vi "Vesta Communication.vi"(8 "error in (no error)":errorcluster, 11 "Message Queues out":T2) -> (0 "error out":errorcluster)   [LabVIEW 2023]
uses:
  Message Queue/All Message Queues.ctl
  Message Queue/Message Cluster.ctl
  Drivers/Resideo Gas Valve/Type Definitions/Vesta Info.ctl
  Drivers/Resideo Gas Valve/Type Definitions/Temperature Control.ctl
  Message Queue/Enqueue Message (Single).vi
  Message Queue/Message Queue.lvlib
panel:
  out "Vesta Data Output":T1
  in  "Debug":bool
  out "Debug":string[](array[string])
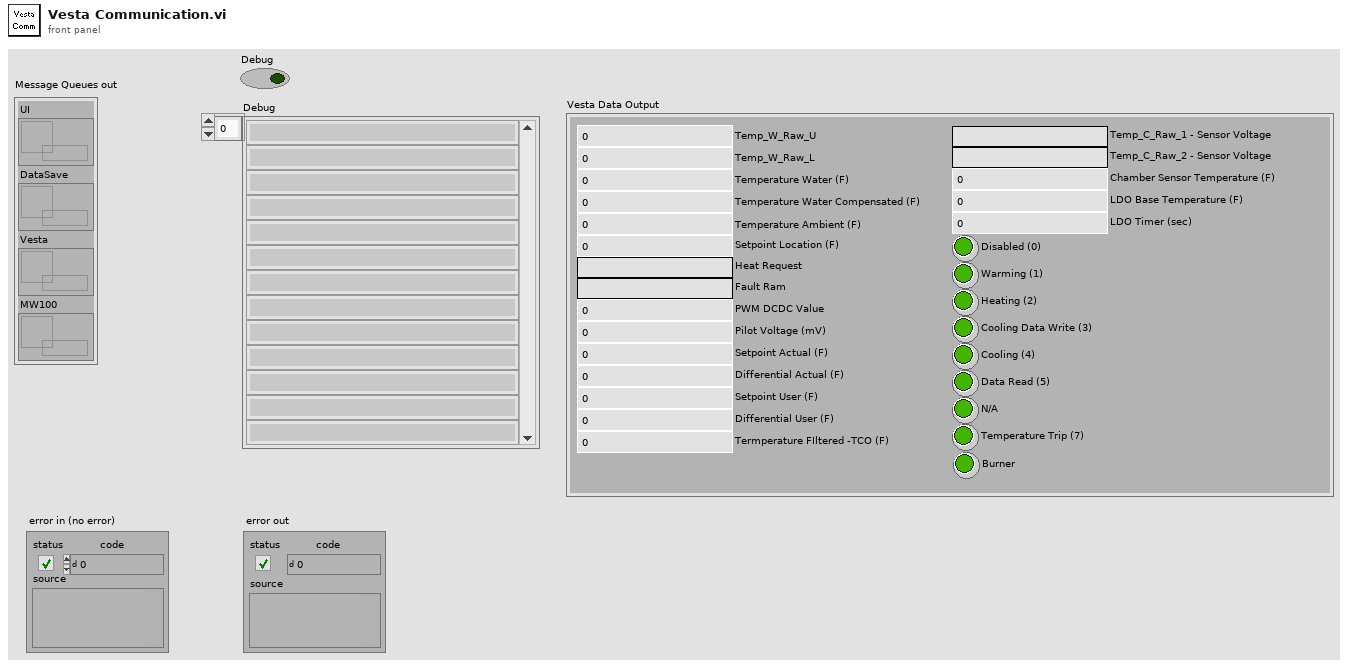
[diagram p1: front panel]
types:
  T1 = typedef "Vesta Info.ctl" = cluster{"Temp_W_Raw_U":u16, "Temp_W_Raw_L":u16, "Temperature Water (F)":dbl, "Temperature Water Compensated (F)":dbl, "Temperature Ambient (F)":dbl, "Setpoint Location (F)":dbl, "Heat Request":string, "Fault Ram":string, "PWM DCDC Value":u16, "Pilot Voltage (mV)":dbl, "Setpoint Actual (F)":dbl, "Differential Actual (F)":dbl, "Setpoint User (F)":dbl, "Differential User (F)":dbl, "Termperature FIltered -TCO (F)":dbl, "Temp_C_Raw_1 - Sensor Voltage":string, "Temp_C_Raw_2 - Sensor Voltage":string, "Chamber Sensor Temperature (F)":dbl, "LDO Base Temperature (F)":dbl, "LDO Timer (sec)":i16, "Disabled (0)":bool, "Warming (1)":bool, "Heating (2)":bool, "Cooling Data Write (3)":bool, "Cooling (4)":bool, "Data Read (5)":bool, "N/A":bool, "Temperature Trip (7)":bool, "Burner":bool}
  T2 = typedef "Message Queue.lvlib/All Message Queues.ctl" = cluster{"UI":refnum<queue>, "DataSave":refnum<queue>, "Vesta":refnum<queue>, "MW100":refnum<queue>}
  T3 = typedef "Temperature Control.ctl" = cluster{"Water Heater Temp (°F)":u16, "Differential  (°F)":dbl}
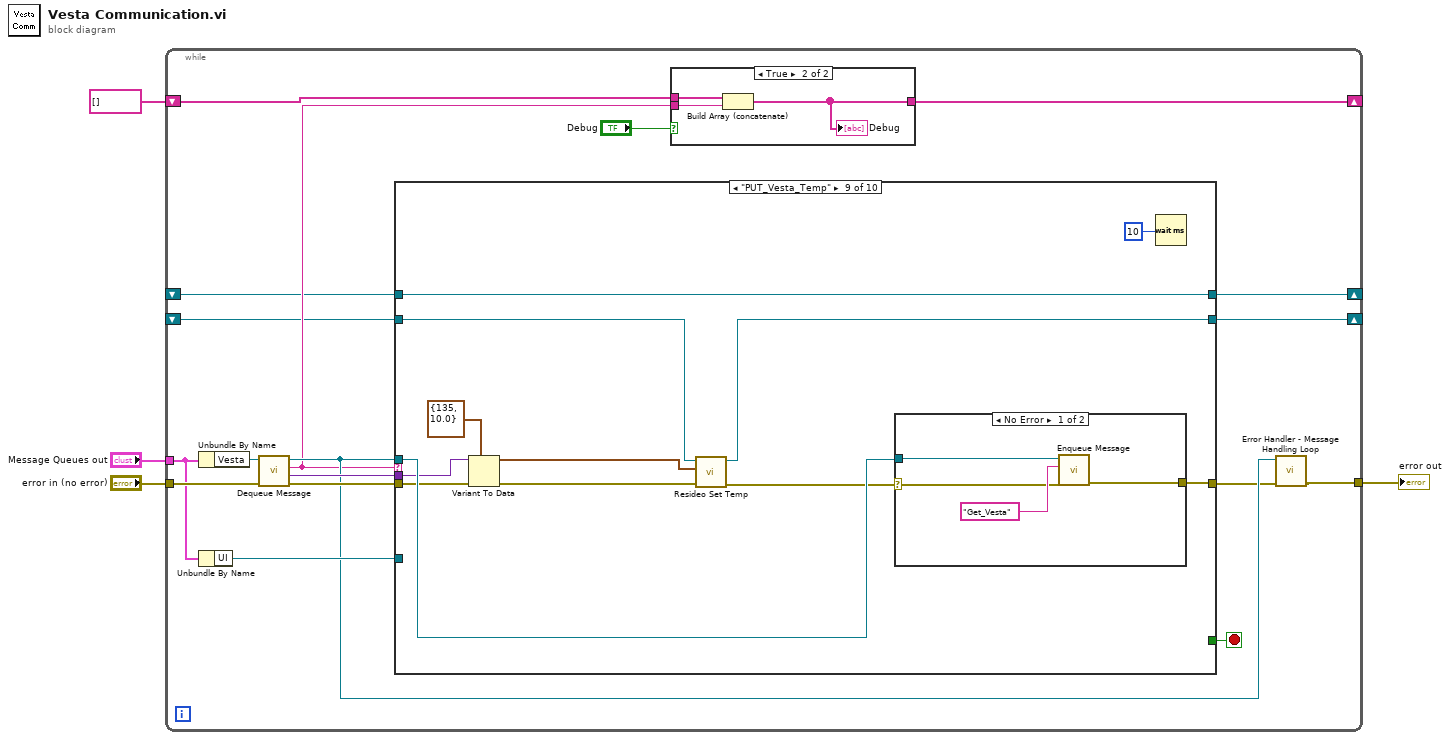
[diagram p0: block diagram]
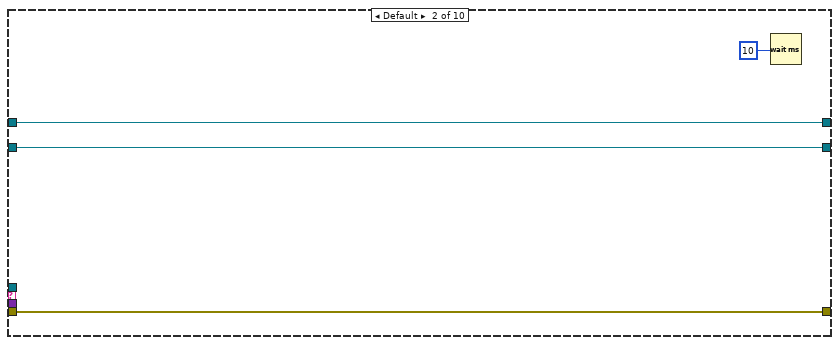
[diagram p4: hidden frame]
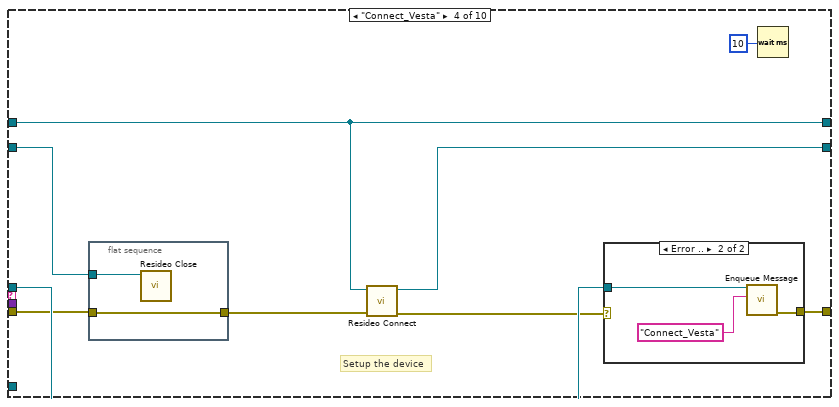
[diagram p6: hidden frame]
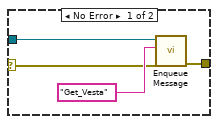
[diagram p7: hidden frame]
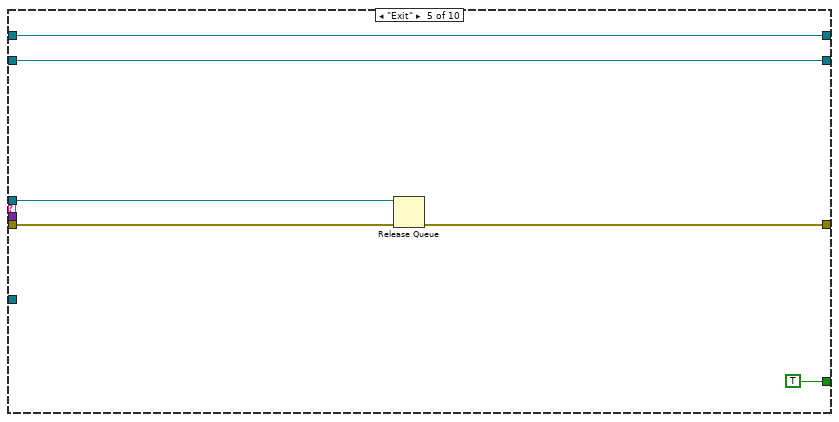
[diagram p8: hidden frame]
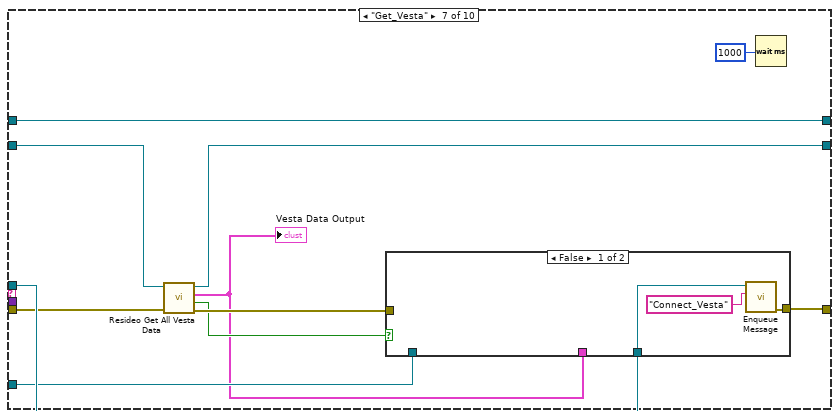
[diagram p10: hidden frame]
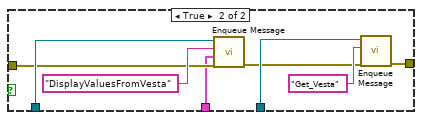
[diagram p11: hidden frame]
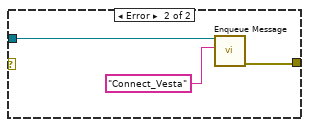
[diagram p13: hidden frame]
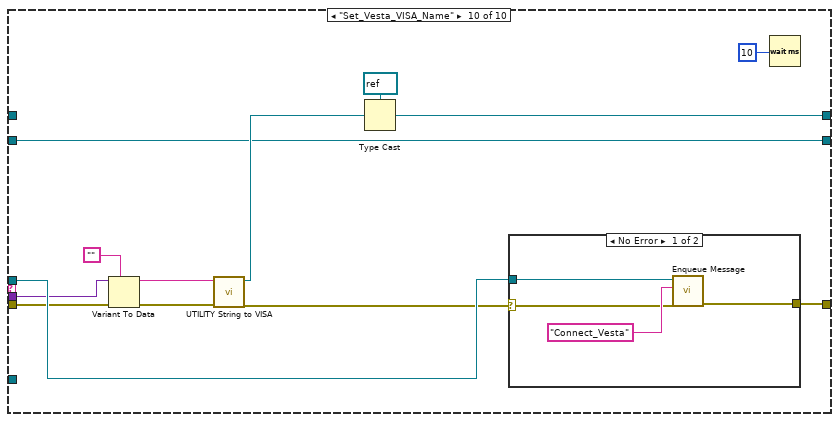
[diagram p14: hidden frame]
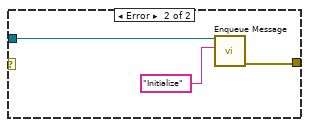
[diagram p15: hidden frame]
diagram:
  n1 = while {
    tunnel: "Message Queues out" -> [w15]
    tunnel: "error in (no error)" -> [w19]
    tunnel: [w11] -> w1
    shift-right: [w16] -> _
    shift-left: string[] [] -> [w17]
    shift-right: [w8] -> _
    shift-left: _ -> [w7]
    shift-right: [w6] -> _
    shift-left: _ -> [w5]
    stop <- w9 stop-if-true
    n2 = Unbundle By Name(w15) -> ("Vesta"=w22:refnum<queue>)
    n3 = Unbundle By Name(w15) -> ("UI"=w14:refnum<queue>)
    n4 = call "Dequeue Message.vi"("error in (no error)"=w19, "Message Queue"=w22) -> ("error out"=w20:errorcluster, "Message Data"=w21:variant, "Message"=w10:string, "dup Message Queue"=w13:refnum<queue>)  [unwired: 6 in]
    n5 = case shown="\"PUT_Vesta_Temp\"" w10 {
      tunnel: w13 -> [_ _ _ w44 w59 _ w73 _ w99 w119]
      tunnel: w21 -> [_ _ _ _ _ _ _ _ w96 w116]
      tunnel: w20 -> [w29 w33 w35 w42 w60 w63 w70 w88 w97 w117]
      tunnel: w14 -> [_ _ _ _ _ _ w72 _ _ _]
      tunnel: [w29 w33 w35 w45 w58 w63 w74 w88 w100 w120] -> w12
      tunnel: [_ _ _ _ TRUE _ _ _ _ _] -> w9
      tunnel: [w28 w32 w36 w38 w56 w62 w68 w87 w89 w109] -> w8
      tunnel: w7 -> [w28 w32 w36 w38 w56 w62 w68 w87 w89 _]
      tunnel: [w27 w31 w34 w39 w55 w61 w67 w86 w90 w108] -> w6
      tunnel: w5 -> [w27 w31 w34 w37 w55 w61 w69 w86 w91 w108]
      frame "---------- Setup ----------" {
      }
      frame Default {
        n6 = Wait (ms)(milliseconds to wait=u32 10) -> ()  [unwired: 1 out]
      }
      frame "Initialize" {
      }
      frame "Connect_Vesta" {
        # "Setup the device"
        n7 = flat-sequence {
          tunnel: w42 -> [w47]
          tunnel: [w47] -> w40
          tunnel: w37 -> [w46]
          frame #0 {
            n8 = call "Resideo Close.vi"("Modbus Master in"=w46) -> ()  [unwired: 10 in, 1 out]
          }
        }
        n9 = call "Resideo Connect.vi"("error in (no error)"=w40, "VISA Refnum in"=w38) -> ("error out"=w41:errorcluster, "Modbus Master out"=w39:refnum<class "Modbus Master.lvclass">)  [unwired: 8 in]
        n10 = case shown="Error .." w41 {
          selector: w41 -> [w48 _]
          tunnel: [w50 w54] -> w45
          tunnel: w44 -> [w49 w52]
          frame No Error {
            n11 = call-poly "Enqueue Message.vi"("error in (no error)"=w48, "Message"="Get_Vesta", "Message Queue"=w49) -> ("error out"=w50:errorcluster)  [unwired: 7 in, 1 out]
          }
          frame Error {
            n12 = call-poly "Enqueue Message.vi"("Message"="Connect_Vesta", "Message Queue"=w52) -> ("error out"=w54:errorcluster)  [unwired: 8 in, 1 out]
          }
        }
        n13 = Wait (ms)(milliseconds to wait=u32 10) -> ()  [unwired: 1 out]
      }
      frame "Exit" {
        n14 = Release Queue(queue=w59, error in (no error)=w60) -> (error out=w58:errorcluster)  [unwired: 1 in, 2 out]
      }
      frame "---------- Data Collection ----------" {
      }
      frame "Get_Vesta" {
        n15 = call "Resideo Get All Vesta Data.vi"("error in (no error)"=w70, "Modbus Master in"=w69) -> ("error out"=w66:errorcluster, "Vesta Is Working"=w65:bool, "Vesta Data Output"=w64:T1, "Modbus Master out"=w67:refnum<class "Modbus Master.lvclass">)  [unwired: 6 in]
        "Vesta Data Output" <- w64
        n16 = case shown="False" w65 {
          tunnel: [w77 w84] -> w74
          tunnel: w73 -> [w75 w83]
          tunnel: w72 -> [_ w81]
          tunnel: w66 -> [_ w79]
          tunnel: w64 -> [_ w78]
          frame False {
            n17 = call-poly "Enqueue Message.vi"("Message"="Connect_Vesta", "Message Queue"=w75) -> ("error out"=w77:errorcluster)  [unwired: 8 in, 1 out]
          }
          frame True {
            n18 = call-poly "Enqueue Message.vi"("error in (no error)"=w79, "Message Data"=w78, "Message"="DisplayValuesFromVesta", "Message Queue"=w81) -> ("error out"=w82:errorcluster)  [unwired: 6 in, 1 out]
            n19 = call-poly "Enqueue Message.vi"("error in (no error)"=w82, "Message"="Get_Vesta", "Message Queue"=w83) -> ("error out"=w84:errorcluster)  [unwired: 7 in, 1 out]
          }
        }
        n20 = Wait (ms)(milliseconds to wait=u32 1000) -> ()  [unwired: 1 out]
      }
      frame "---------- Timer Control ----------" {
      }
      frame "PUT_Vesta_Temp" {
        n21 = Variant To Data(error in=w97, type=T3 {"Water Heater Temp (°F)"=135, "Differential  (°F)"=10.0} ("Temperature Parameters"), Variant=w96) -> (data=w92:T3, error out=w94:errorcluster)
        n22 = call "Resideo Set Temp.vi"("error in (no error)"=w94, "Vesta Data"=w92, "Modbus Master in"=w91) -> ("error out"=w93:errorcluster, "Modbus Master out"=w90:refnum<class "Modbus Master.lvclass">)  [unwired: 7 in]
        n23 = case shown="No Error" w93 {
          selector: w93 -> [w101 _]
          tunnel: [w103 w107] -> w100
          tunnel: w99 -> [w102 w105]
          frame No Error {
            n24 = call-poly "Enqueue Message.vi"("error in (no error)"=w101, "Message"="Get_Vesta", "Message Queue"=w102) -> ("error out"=w103:errorcluster)  [unwired: 7 in, 1 out]
          }
          frame Error {
            n25 = call-poly "Enqueue Message.vi"("Message"="Connect_Vesta", "Message Queue"=w105) -> ("error out"=w107:errorcluster)  [unwired: 8 in, 1 out]
          }
        }
        n26 = Wait (ms)(milliseconds to wait=u32 10) -> ()  [unwired: 1 out]
      }
      frame "Set_Vesta_VISA_Name" {
        n27 = Variant To Data(error in=w117, type="", Variant=w116) -> (data=w110:string, error out=w112:errorcluster)
        n28 = call "UTILITY String to VISA.vi"("error in (no error)"=w112, "VISA Name"=w110) -> ("error out"=w111:errorcluster, "VISA resource name out"=w113:refnum<visa-resource-name>)  [unwired: 8 in]
        n29 = Type Cast(type=refnum<visa-resource-name> refnum ("VISA Refnum in"), x=w113) -> (*(type *) &x=w109:refnum<visa-resource-name>)
        n30 = case shown="No Error" w111 {
          selector: w111 -> [w121 _]
          tunnel: [w123 w127] -> w120
          tunnel: w119 -> [w122 w125]
          frame No Error {
            n31 = call-poly "Enqueue Message.vi"("error in (no error)"=w121, "Message"="Connect_Vesta", "Message Queue"=w122) -> ("error out"=w123:errorcluster)  [unwired: 7 in, 1 out]
          }
          frame Error {
            n32 = call-poly "Enqueue Message.vi"("Message"="Initialize", "Message Queue"=w125) -> ("error out"=w127:errorcluster)  [unwired: 8 in, 1 out]
          }
        }
        n33 = Wait (ms)(milliseconds to wait=u32 10) -> ()  [unwired: 1 out]
      }
    }
    n34 = case shown="True" "Debug" {
      tunnel: w10 -> [_ w26]
      tunnel: w17 -> [w23 w25]
      tunnel: [w23 w24] -> w16
      frame False {
      }
      frame True {
        n35 = Build Array (concatenate)(w25, w26) -> (w24:string[])
        "Debug" <- w24
      }
    }
    n36 = call "Error Handler - Message Handling Loop.vi"("error in (no error)"=w12, "Message Queue"=w13) -> ("dup error in"=w11:errorcluster)  [unwired: 8 in, 1 out]
  }
  "error out" <- w1
